vi "Ex. 3. Acquire Data from Device.vi"() -> ()   [LabVIEW 2024]
uses:
  <vilib>/DAQmx/read.llb/DAQmx Read (Analog Wfm 1Chan NSamp).vi
  <vilib>/DAQmx/create/channels.llb/DAQmx Create Channel (AI-Voltage-Basic).vi
  <vilib>/DAQmx/configure/timing.llb/DAQmx Timing (Sample Clock).vi
  <vilib>/DAQmx/miscellaneous.llb/DAQmx Fill In Error Info.vi
  <vilib>/measure/maspectr.llb/FFT Power Spectrum and PSD for 1 Chan.vi
  <vilib>/measure/NI_MAPro.lvlib
panel:
  in  "Voltage Input":tag
  in  "File Path":path
  out "Frequency Domain Signal":cluster{"f0":dbl, "df":dbl, "magnitude":dbl[]}(graph)
  in  "Stop":bool
  out "Time-Domain Signal":waveform(dbl)(graph)
  # "Acquire Data from Device"
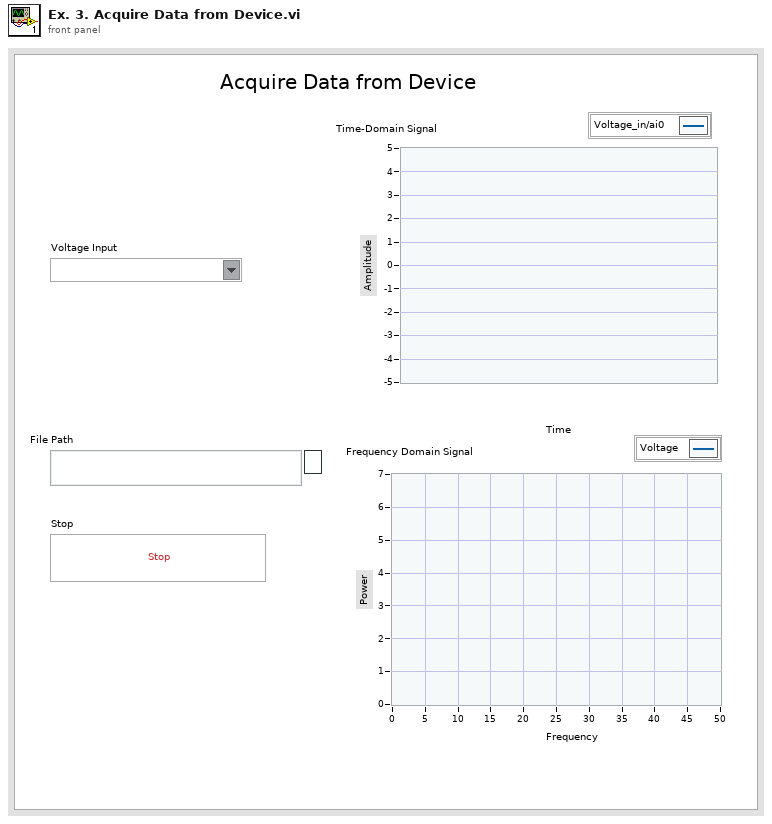
[diagram p1: front panel]
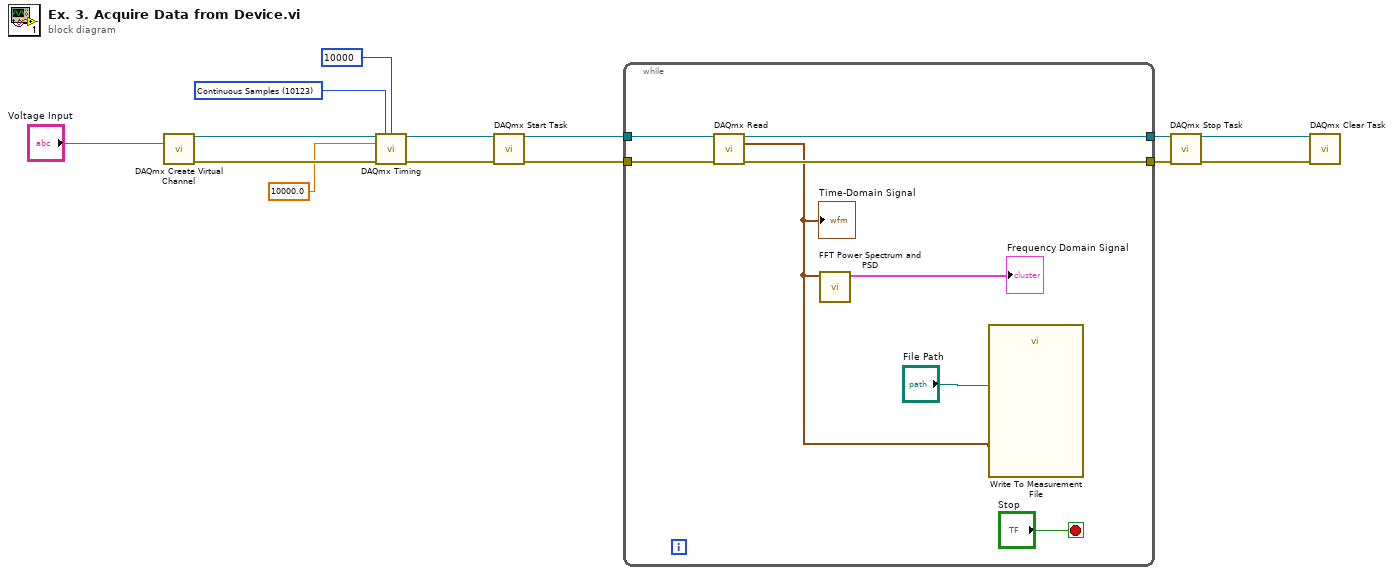
[diagram p0: block diagram]
diagram:
  w2 = 10123 items=["Finite Samples"=10178, "Continuous Samples"=10123, "Hardware Timed Single Point"=12522] ("sample mode")
  n1 = call-poly <vilib>:"DAQmx Create Virtual Channel.vi"("physical channels"="Voltage Input") -> ("task out"=w13:refnum<k21>, "error out"=w12:errorcluster)  [unwired: 13 in]
  n2 = call-poly <vilib>:"DAQmx Timing.vi"("task/channels in"=w13, "sample mode"=w2, "samples per channel"=10000, "rate"=10000.0, "error in"=w12) -> ("task out"=w11:refnum<k21>, "error out"=w10:errorcluster)  [unwired: 9 in]
  n3 = call <vilib>:"DAQmx Start Task.vi"("task/channels in"=w11, "error in"=w10) -> ("task out"=w9:refnum<k21>, "error out"=w8:errorcluster)  [unwired: 12 in]
  n4 = while {
    tunnel: w9 -> [w19]
    tunnel: w8 -> [w18]
    tunnel: [w17] -> w7
    tunnel: [w16] -> w6
    stop <- "Stop" stop-if-true
    n5 = call-poly <vilib>:"DAQmx Read.vi"("task/channels in"=w19, "error in"=w18) -> ("task out"=w17:refnum<k21>, "data"=w15:waveform(dbl), "error out"=w16:errorcluster)  [unwired: 11 in]
    "Time-Domain Signal" <- w15
    n6 = call-poly <vilib>:"FFT Power Spectrum and PSD.vi"("time signal"=w15) -> ("Power Spectrum / PSD"=→"Frequency Domain Signal":cluster{"f0":dbl, "df":dbl, "magnitude":dbl[]})  [unwired: 7 in, 3 out]
    n7 = call "Write To Measurement File"("Signals"=w15, "Filename"="File Path") -> ()  [unwired: 15 in, 3 out]
  }
  n8 = call <vilib>:"DAQmx Stop Task.vi"("task/channels in"=w7, "error in"=w6) -> ("task out"=w5:refnum<k21>, "error out"=w4:errorcluster)  [unwired: 12 in]
  n9 = call <vilib>:"DAQmx Clear Task.vi"("task in"=w5, "error in"=w4) -> ()  [unwired: 13 in, 1 out]
